vi "DRIVE ROBOT TELEOP.vi"(6 "TURBO":cluster{"button":i32, "%speed":dbl}={"button"=2, "%speed"=1.0} {"%speed" min=0.0 max=1.0 format="%.3g"}, 9 "TURTLE":cluster{"button":i32, "%speed":dbl}={"button"=4, "%speed"=0.5} {"%speed" min=0.0 max=1.0 format="%.3g"}, 10 "NORMAL":cluster{"button":i32, "%speed":dbl}={"button"=0, "%speed"=0.75} {"%speed" min=0.0 max=1.0 format="%.3g"}, 11 "Joystick values":T1(array[cluster])) -> ()   [LabVIEW 2020]
uses:
  <vilib>/Rock Robotics/Network Tables/NT Read Boolean.vi
  Robot Global Data.vi
  <vilib>/Rock Robotics/WPI/Utilities/WPI_GetSetVariantRefNum.vi
  <vilib>/Rock Robotics/Network Tables/NT Write Numeric Array.vi
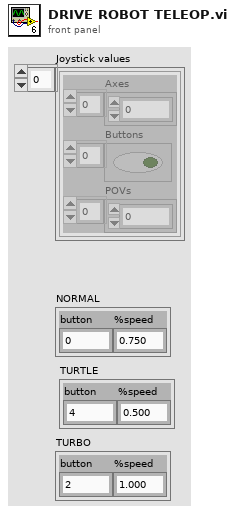
[diagram p1: front panel]
types:
  T1 = cluster{"Axes":dbl[], "Buttons":bool[], "POVs":i16[]}[]
  T2 = cluster{"Axes":dbl[], "Buttons":bool[], "POVs":i16[]}
  T3 = typedef "WPI_RobotDriveDevRef.ctl" = cluster{"DevStatus":errorcluster, "Motors[]":T4[], "Square Inputs":bool, "Max Output":dbl}
  T4 = typedef "WPI_MotorControlDeviceRef.ctl" = cluster{"DeviceStatus":errorcluster, "Type":T5, "PWM":cluster{"PWM Channel":T6, "DeadBand":T7}, "CAN":cluster{"Device Number":u8, "SetOutput VI Ref":variant, "GetOutput VI Ref":variant, "Enable VI Ref":variant, "Disable VI Ref":variant, "Data":variant}, "Invert":bool, "DIO PWM":cluster{"PWM \"Enable\" Channel":T6, "DIOChannel":T8, "PWM Rate":dbl}}
  T5 = typedef "WPI_MotorControlType.ctl" = enum16{"PWM", "CAN", "DIO PWM"}
  T6 = typedef "FPGA_DIOPWMChannel.ctl" = enum8{"PWM 0", "PWM 1", "PWM 2", "PWM 3", "PWM 4", "PWM 5", "PWM 6", "PWM 7", "PWM 8", "PWM 9", "PWM MXP 0", "PWM MXP 1", "PWM MXP 2", "PWM MXP 3", "PWM MXP 4", "PWM MXP 5", "PWM MXP 6", "PWM MXP 7", "PWM MXP 8", "PWM MXP 9", "Invalid"}
  T7 = typedef "WPI_PWMDeadband.ctl" = cluster{"Name":string, "maxPositivePwm":i32, "minPositivePwm":i32, "centerPwm":i32, "maxNegativePwm":i32, "minNegativePwm":i32, "angularRange":u16}
  T8 = typedef "FPGA_DIOChannel.ctl" = enum8{"DIO 0", "DIO 1", "DIO 2", "DIO 3", "DIO 4", "DIO 5", "DIO 6", "DIO 7", "DIO 8", "DIO 9", "DIO MXP 0", "DIO MXP 1", "DIO MXP 2", "DIO MXP 3", "DIO MXP 4", "DIO MXP 5", "DIO MXP 6", "DIO MXP 7", "DIO MXP 8", "DIO MXP 9", "DIO MXP 10", "DIO MXP 11", "DIO MXP 12", "DIO MXP 13", "DIO MXP 14", "DIO MXP 15", "SPI Port CS1", "SPI Port CS2", "SPI Port CS3", "SPI Port MISO", "SPI Port MOSI", "Invalid"}
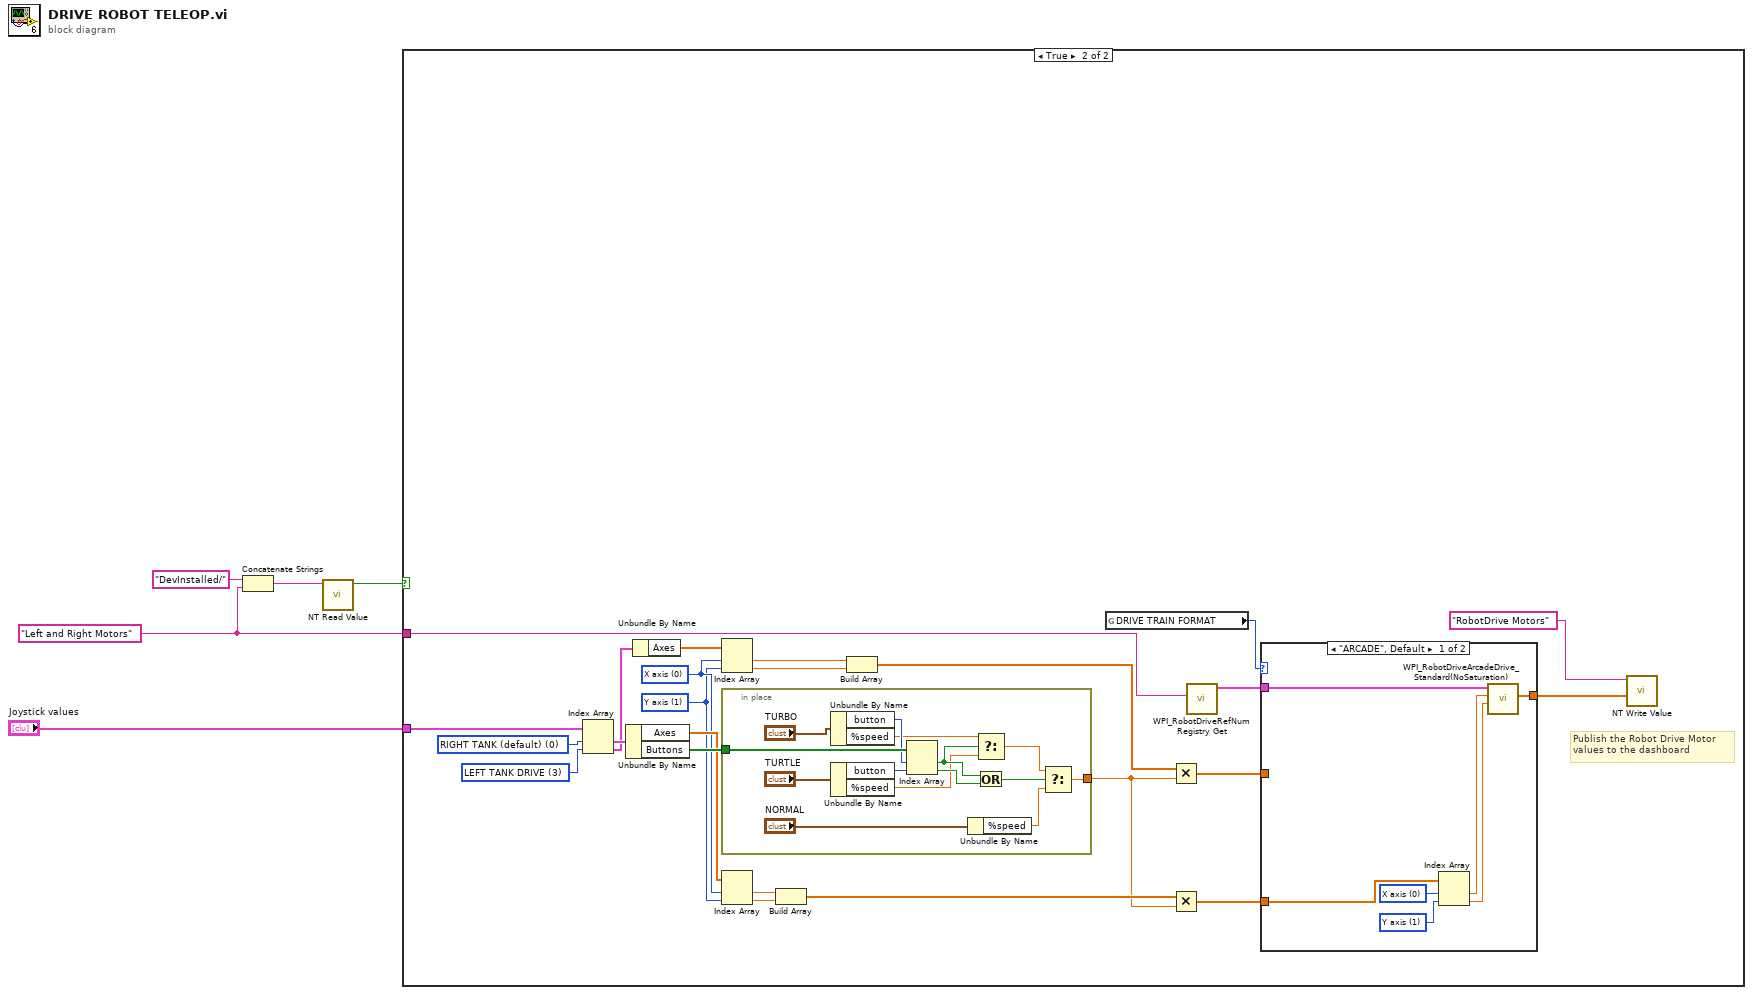
[diagram p0: block diagram]
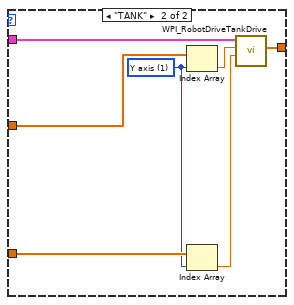
[diagram p3: hidden frame]
diagram:
  w4 = "Left and Right Motors" ("Name")
  n1 = Concatenate Strings("DevInstalled/" ("Name"), w4) -> (w2:string)
  n2 = call-poly <vilib>:"NT Read Value.vi"("Name"=w2) -> ("Boolean"=w1:bool)  [unwired: 9 in, 1 out]
  n3 = case shown="True" w1 {
    tunnel: w4 -> [_ w26]
    tunnel: "Joystick values" -> [_ w15]
    frame False {
    }
    frame True {
      w6 = u16 3 items=["RIGHT TANK (default)", "LEFT ARM", "RIGHT ARM", "LEFT TANK DRIVE"] ("Joysticks")
      w7 = u16 0 items=["RIGHT TANK (default)", "LEFT ARM", "RIGHT ARM", "LEFT TANK DRIVE"] ("Joysticks")
      w8 = u16 1 items=["X axis", "Y axis", "Z axis"] ("AXIS VALUES")
      w9 = u16 0 items=["X axis", "Y axis", "Z axis"] ("AXIS VALUES")
      # "Publish the Robot Drive Motor\nvalues to the dashboard"
      n4 = Index Array(array=w15, index #1=w7, index #2=w6) -> (element #1=w14:T2, element #2=w11:T2)
      n5 = Unbundle By Name(w14) -> ("Axes"=w12:dbl[], "Buttons"=w13:bool[])
      n6 = Unbundle By Name(w11) -> ("Axes"=w10:dbl[])
      n7 = Index Array(array=w10, index #1=w9, index #2=w8) -> (element #1=w23:dbl, element #2=w22:dbl)
      n8 = in-place {
        in-place-border: w13 -> [w57]
        in-place-border: [w52] -> w16
        n9 = Unbundle By Name("TURBO") -> ("button"=w55:i32, "%speed"=w47:dbl)
        n10 = Unbundle By Name("TURTLE") -> ("button"=w53:i32, "%speed"=w46:dbl)
        n11 = Index Array(array=w57, index #1=w55, index #2=w53) -> (element #1=w48:bool, element #2=w50:bool)
        n12 = Unbundle By Name("NORMAL") -> ("%speed"=w44:dbl)
        n13 = Select(t=w47, s=w48, f=w46) -> (s? t:f=w49:dbl)
        n14 = Or(x=w48, y=w50) -> (x .or. y?=w51:bool)
        n15 = Select(t=w49, s=w51, f=w44) -> (s? t:f=w52:dbl)
      }
      n16 = Index Array(array=w12, index #1=w9, index #2=w8) -> (element #1=w25:dbl, element #2=w24:dbl)
      n17 = Build Array(w25, w24) -> (w19:dbl[])
      n18 = Build Array(w23, w22) -> (w20:dbl[])
      n19 = global read "Robot Global Data.vi" "DRIVE TRAIN FORMAT"() -> (w21:enum16{"ARCADE", "TANK"})
      n20 = Multiply(x=w20, y=w16) -> (x*y=w17:dbl[])
      n21 = Multiply(x=w19, y=w16) -> (x*y=w18:dbl[])
      n22 = call <vilib>:"WPI_RobotDriveRefNum Registry Get.vi"("refnum name"=w26) -> ("RobotDriveDevRef"=w29:T3)  [unwired: 1 in, 9 out]
      n23 = case shown="\"ARCADE\", Default" w21 {
        tunnel: w29 -> [w36 w42]
        tunnel: [w35 w43] -> w28
        tunnel: w17 -> [_ w41]
        tunnel: w18 -> [w32 w39]
        frame "ARCADE", Default {
          w31 = u16 0 items=["X axis", "Y axis", "Z axis"] ("AXIS VALUES")
          w30 = u16 1 items=["X axis", "Y axis", "Z axis"] ("AXIS VALUES")
          n24 = Index Array(array=w32, index #1=w31, index #2=w30) -> (element #1=w34:dbl, element #2=w33:dbl)
          n25 = call <vilib>:"WPI_RobotDriveArcadeDrive_Standard(NoSaturation).vi"("Y axis value"=w33, "X axis value"=w34, "RobotDriveDevRef"=w36) -> ("Motor Values"=w35:dbl[])  [unwired: 1 in, 7 out]
        }
        frame "TANK" {
          w37 = u16 1 items=["X axis", "Y axis", "Z axis"] ("AXIS VALUES")
          n26 = Index Array(array=w41, index=w37) -> (element=w40:dbl)
          n27 = Index Array(array=w39, index=w37) -> (element=w38:dbl)
          n28 = call <vilib>:"WPI_RobotDriveTankDrive.vi"("Right axis value"=w38, "Left axis value"=w40, "RobotDriveDevRef"=w42) -> ("Motor Values"=w43:dbl[])  [unwired: 6 in, 2 out]
        }
      }
      n29 = call-poly <vilib>:"NT Write Value.vi"("Numeric Array"=w28, "Name"="RobotDrive Motors") -> ()  [unwired: 9 in, 1 out]
    }
  }
